vi "osciloscope-4-chan.vi"(0 "COM Port":refnum<visa-resource-name>, 5 "Baud Rate (BPS)":u32=9600, 7 "Sampling Frequency (Hz)":sgl, 9 "Refresh Button":bool, 11 "Stop Button":bool, 12 "Time Domain (Block Size)":u16(knob) scale=4.0..10.0, 13 "Frequency Domain (Block Size)":u16(knob) scale=4.0..10.0, 14 "Decimation Factor":u8=1 min=1 max=100) -> (4 "Time Domain":waveform(dbl)[](graph), 6 "Frequency Domain":cluster{"f0":dbl, "df":dbl, "magnitude":dbl[]}[](graph))   [LabVIEW 2023]
uses:
  <vilib>/Analysis/2dsp.llb/Decimate (single shot, DBL).vi
  <vilib>/Instr/_visa.llb/VISA Configure Serial Port (Instr).vi
  <vilib>/express/express analysis/Spectral/Block/exnSpectralBlock spectral measurements peak poly.vi
  <vilib>/express/express analysis/Spectral/Block/exnSpectralBlock spectral measurements peak WFM.vi
  <vilib>/express/express analysis/Spectral/XNode/ExpressSpectralMeasurementsBlockNode.xnode
  <vilib>/Analysis/NI_AALPro.lvlib
panel:
  out "Frerquency Domain Indicator":u32
  out "Time Domain Indicator":u32
  # "4-CHANNEL OSCILOSCOPE"
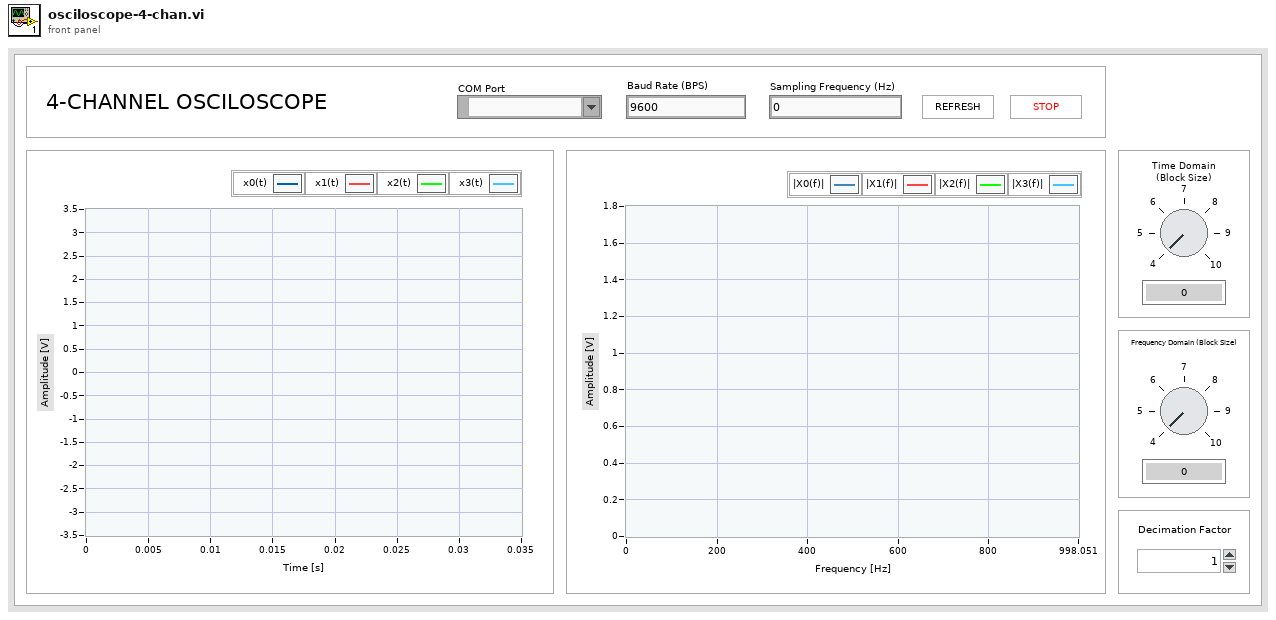
[diagram p1: front panel]
types:
  T1 = cluster{"averaging mode":u16, "weighting mode":u16, "number of averages":u32}
  T2 = cluster{"dB On (F)":bool, "unwrap phase (F)":bool, "convert to degree (F)":bool}
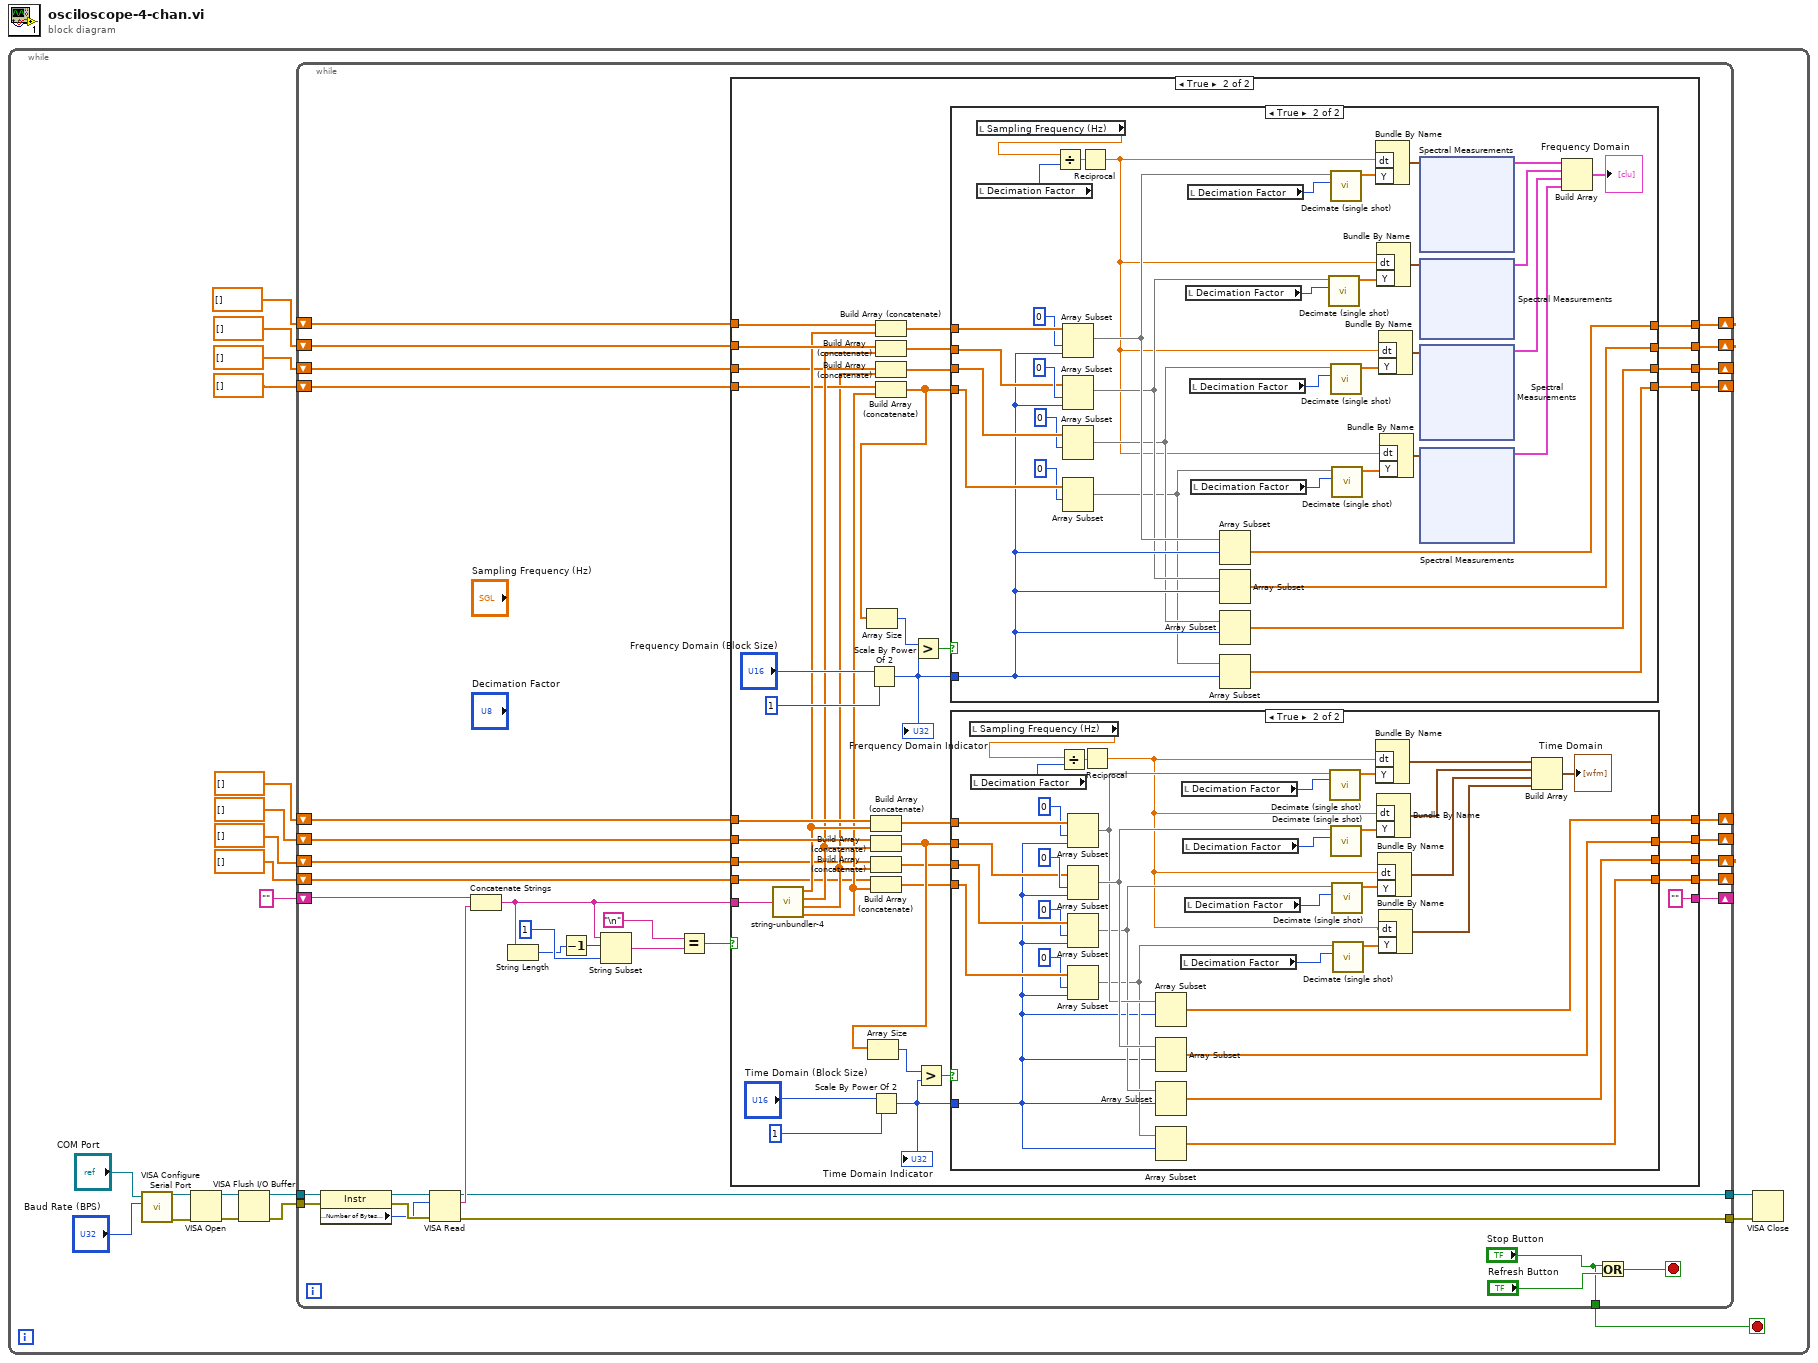
[diagram p0: block diagram]
diagram:
  n1 = while {
    stop <- w9 stop-if-true
    n2 = call-poly "VISA Configure Serial Port"("VISA resource name"="COM Port", "baud rate (9600)"="Baud Rate (BPS)") -> ("VISA resource name out"=w18:refnum<visa-resource-name>, "error out"=w19:errorcluster)  [unwired: 12 in]
    n3 = VISA Open(error in (no error)=w19, VISA resource name=w18) -> (VISA resource name=w17:refnum<visa-resource-name>, error out=w16:errorcluster)  [unwired: 3 in]
    n4 = VISA Flush I/O Buffer(VISA resource name=w17, error in (no error)=w16) -> (VISA resource name out=w20:refnum<visa-resource-name>, error out=w13:errorcluster)  [unwired: 1 in]
    n5 = while {
      tunnel: w20 -> [w56]
      tunnel: w13 -> [w55]
      tunnel: [w36] -> w12
      tunnel: [w37] -> w11
      shift-right: [w49] -> _
      shift-left: "" -> [w50]
      shift-right: [w39] -> _
      shift-left: dbl[] [] -> [w40]
      shift-right: [w38] -> _
      shift-left: dbl[] [] -> [w41]
      shift-right: [w33] -> _
      shift-left: dbl[] [] -> [w35]
      shift-right: [w32] -> _
      shift-left: dbl[] [] -> [w34]
      tunnel: ["Stop Button"] -> w9
      shift-right: [w28] -> _
      shift-left: dbl[] [] -> [w26]
      shift-right: [w27] -> _
      shift-left: dbl[] [] -> [w25]
      shift-right: [w24] -> _
      shift-left: dbl[] [] -> [w22]
      shift-right: [w23] -> _
      shift-left: dbl[] [] -> [w21]
      stop <- w31 stop-if-true
      n6 = property class="Instr"(reference=w56, error in=w55) -> (reference out=w54:refnum<visa-resource-name>, error out=w53:errorcluster, "Serial Settings:Number of Bytes at Serial Port"=w52:u32)
      n7 = VISA Read(VISA resource name=w54, byte count=w52, error in (no error)=w53) -> (VISA resource name out=w37:refnum<visa-resource-name>, read buffer=w51:string, error out=w36:errorcluster)  [unwired: 1 out]
      n8 = Concatenate Strings(w50, w51) -> (w47:string)
      n9 = String Length(string=w47) -> (length=w45:i32)
      n10 = Decrement(x=w45) -> (x-1=w46:i32)
      n11 = String Subset(string=w47, offset (0)=w46, length (rest)=1 ("length (rest)")) -> (substring=w43:string)
      n12 = Equal?(x="\n", y=w43) -> (x = y?=w42:bool)
      n13 = case shown="True" w42 {
        tunnel: w41 -> [w64 w104]
        tunnel: w47 -> [w65 w81]
        tunnel: [w65 ""] -> w49
        tunnel: w40 -> [w63 w102]
        tunnel: [w63 w99] -> w39
        tunnel: [w64 w100] -> w38
        tunnel: w35 -> [w62 w96]
        tunnel: w34 -> [w61 w95]
        tunnel: [w62 w94] -> w33
        tunnel: [w61 w93] -> w32
        tunnel: [w60 w78] -> w28
        tunnel: [w59 w77] -> w27
        tunnel: w26 -> [w60 w76]
        tunnel: w25 -> [w59 w75]
        tunnel: [w58 w72] -> w24
        tunnel: [w57 w71] -> w23
        tunnel: w22 -> [w58 w68]
        tunnel: w21 -> [w57 w67]
        frame False {
        }
        frame True {
          n14 = call "string-unbundler-4.vi"("String"=w81) -> ("Array 1"=w80:dbl[], "Array 2"=w79:dbl[], "Array 3"=w74:dbl[], "Array 4"=w73:dbl[])
          n15 = Scale By Power Of 2(n="Frequency Domain (Block Size)", x=u32 1) -> (x*2^n=w87:u32)
          "Frerquency Domain Indicator" <- w87
          n16 = Build Array (concatenate)(w104, w80) -> (w92:dbl[])
          n17 = Build Array (concatenate)(w102, w79) -> (w98:dbl[])
          n18 = Array Size(array=w98) -> (size(s)=w105:i32)
          n19 = Build Array (concatenate)(w68, w74) -> (w70:dbl[])
          n20 = Build Array (concatenate)(w67, w73) -> (w69:dbl[])
          n21 = Scale By Power Of 2(n="Time Domain (Block Size)", x=u32 1) -> (x*2^n=w84:u32)
          "Time Domain Indicator" <- w84
          n22 = Build Array (concatenate)(w96, w80) -> (w97:dbl[])
          n23 = Build Array (concatenate)(w95, w79) -> (w90:dbl[])
          n24 = Build Array (concatenate)(w76, w74) -> (w82:dbl[])
          n25 = Build Array (concatenate)(w75, w73) -> (w66:dbl[])
          n26 = Array Size(array=w66) -> (size(s)=w89:i32)
          n27 = Greater?(x=w89, y=w87) -> (0:w91:bool)
          n28 = Greater?(x=w105, y=w84) -> (0:w101:bool)
          n29 = case shown="True" w91 {
            tunnel: w97 -> [w109 w147]
            tunnel: w90 -> [w108 w144]
            tunnel: w87 -> [_ w123]
            tunnel: [w109 w143] -> w94
            tunnel: [w108 w142] -> w93
            tunnel: w82 -> [w107 w127]
            tunnel: w66 -> [w106 w125]
            tunnel: [w107 w112] -> w78
            tunnel: [w106 w111] -> w77
            frame False {
            }
            frame True {
              n30 = local read "Sampling Frequency (Hz)"() -> (w132:sgl)
              n31 = local read "Decimation Factor"() -> (w133:u8)
              n32 = Divide(x=w132, y=w133) -> (x/y=w134:sgl)
              n33 = Array Subset(array=w147, index=0, length=w123) -> (w116:dbl[])
              n34 = Array Subset(array=w144, index=0, length=w123) -> (w115:dbl[])
              n35 = Array Subset(array=w127, index=0) -> (w114:dbl[])  [unwired: 1 in]
              n36 = Array Subset(array=w125, index=0) -> (w113:dbl[])  [unwired: 1 in]
              n37 = Reciprocal(x=w134) -> (1/x=w110:sgl)
              n38 = local read "Decimation Factor"() -> (w130:u8)
              n39 = local read "Decimation Factor"() -> (w131:u8)
              n40 = local read "Decimation Factor"() -> (w118:u8)
              n41 = local read "Decimation Factor"() -> (w117:u8)
              n42 = Array Subset(array=w116, index=w123) -> (w143:dbl[])  [unwired: 1 in]
              n43 = Array Subset(array=w115, index=w123) -> (w142:dbl[])  [unwired: 1 in]
              n44 = Array Subset(array=w114, index=w123) -> (w112:dbl[])  [unwired: 1 in]
              n45 = Array Subset(array=w113, index=w123) -> (w111:dbl[])  [unwired: 1 in]
              n46 = call-poly <vilib>:"Decimate (single shot).vi"("decimating factor"=w130, "X"=w115) -> ("Decimated Array"=w136:dbl[])  [unwired: 8 in, 1 out]
              n47 = call-poly <vilib>:"Decimate (single shot).vi"("decimating factor"=w131, "X"=w116) -> ("Decimated Array"=w135:dbl[])  [unwired: 8 in, 1 out]
              n48 = call-poly <vilib>:"Decimate (single shot).vi"("decimating factor"=w118, "X"=w114) -> ("Decimated Array"=w120:dbl[])  [unwired: 8 in, 1 out]
              n49 = call-poly <vilib>:"Decimate (single shot).vi"("decimating factor"=w117, "X"=w113) -> ("Decimated Array"=w119:dbl[])  [unwired: 8 in, 1 out]
              n50 = Bundle By Name("dt"=w110, "Y"=w135) -> (w137:waveform(dbl))  [unwired: 1 in]
              n51 = Bundle By Name("dt"=w110, "Y"=w136) -> (w138:waveform(dbl))  [unwired: 1 in]
              n52 = Bundle By Name("dt"=w110, "Y"=w120) -> (w121:waveform(dbl))  [unwired: 1 in]
              n53 = Bundle By Name("dt"=w110, "Y"=w119) -> (w122:waveform(dbl))  [unwired: 1 in]
              n54 = xnode "Spectral Measurements"("Signals"=w137) -> ("FFT - (Peak)"=w139:cluster{"f0":dbl, "df":dbl, "magnitude":dbl[]})  [unwired: 1 in, 2 out]
              n55 = xnode "Spectral Measurements"("Signals"=w138) -> ("FFT - (Peak)"=w140:cluster{"f0":dbl, "df":dbl, "magnitude":dbl[]})  [unwired: 1 in, 2 out]
              n56 = xnode "Spectral Measurements"("Signals"=w121) -> ("FFT - (Peak)"=w129:cluster{"f0":dbl, "df":dbl, "magnitude":dbl[]})  [unwired: 1 in, 2 out]
              n57 = xnode "Spectral Measurements"("Signals"=w122) -> ("FFT - (Peak)"=w128:cluster{"f0":dbl, "df":dbl, "magnitude":dbl[]})  [unwired: 1 in, 2 out]
              n58 = Build Array(w139, w140, w129, w128) -> (→"Frequency Domain":cluster{"f0":dbl, "df":dbl, "magnitude":dbl[]}[])
            }
          }
          n59 = case shown="True" w101 {
            tunnel: w92 -> [w191 w225]
            tunnel: w98 -> [w190 w223]
            tunnel: w84 -> [_ w195]
            tunnel: [w191 w219] -> w100
            tunnel: [w190 w218] -> w99
            tunnel: [w188 w201] -> w71
            tunnel: [w189 w200] -> w72
            tunnel: w70 -> [w189 w199]
            tunnel: w69 -> [w188 w198]
            frame False {
            }
            frame True {
              n60 = local read "Sampling Frequency (Hz)"() -> (w211:sgl)
              n61 = local read "Decimation Factor"() -> (w212:u8)
              n62 = Divide(x=w211, y=w212) -> (x/y=w210:sgl)
              n63 = Array Subset(array=w225, index=0, length=w195) -> (w215:dbl[])
              n64 = Array Subset(array=w223, index=0, length=w195) -> (w217:dbl[])
              n65 = Array Subset(array=w199, index=0, length=w195) -> (w203:dbl[])
              n66 = Array Subset(array=w198, index=0, length=w195) -> (w202:dbl[])
              n67 = Reciprocal(x=w210) -> (1/x=w192:sgl)
              n68 = Array Subset(array=w215, index=w195) -> (w219:dbl[])  [unwired: 1 in]
              n69 = Array Subset(array=w217, index=w195) -> (w218:dbl[])  [unwired: 1 in]
              n70 = Array Subset(array=w203, index=w195) -> (w200:dbl[])  [unwired: 1 in]
              n71 = Array Subset(array=w202, index=w195) -> (w201:dbl[])  [unwired: 1 in]
              n72 = local read "Decimation Factor"() -> (w193:u8)
              n73 = local read "Decimation Factor"() -> (w209:u8)
              n74 = local read "Decimation Factor"() -> (w208:u8)
              n75 = local read "Decimation Factor"() -> (w194:u8)
              n76 = call-poly <vilib>:"Decimate (single shot).vi"("decimating factor"=w209, "X"=w215) -> ("Decimated Array"=w214:dbl[])  [unwired: 8 in, 1 out]
              n77 = call-poly <vilib>:"Decimate (single shot).vi"("decimating factor"=w208, "X"=w217) -> ("Decimated Array"=w216:dbl[])  [unwired: 8 in, 1 out]
              n78 = call-poly <vilib>:"Decimate (single shot).vi"("decimating factor"=w194, "X"=w203) -> ("Decimated Array"=w206:dbl[])  [unwired: 8 in, 1 out]
              n79 = call-poly <vilib>:"Decimate (single shot).vi"("decimating factor"=w193, "X"=w202) -> ("Decimated Array"=w207:dbl[])  [unwired: 8 in, 1 out]
              n80 = Bundle By Name("dt"=w192, "Y"=w214) -> (w220:waveform(dbl))  [unwired: 1 in]
              n81 = Bundle By Name("dt"=w192, "Y"=w216) -> (w221:waveform(dbl))  [unwired: 1 in]
              n82 = Bundle By Name("dt"=w192, "Y"=w206) -> (w205:waveform(dbl))  [unwired: 1 in]
              n83 = Bundle By Name("dt"=w192, "Y"=w207) -> (w204:waveform(dbl))  [unwired: 1 in]
              n84 = Build Array(w220, w221, w205, w204) -> (→"Time Domain":waveform(dbl)[])
            }
          }
        }
      }
      n85 = Or(x="Stop Button", y="Refresh Button") -> (x .or. y?=w31:bool)
    }
    n86 = VISA Close(VISA resource name=w11, error in (no error)=w12) -> ()  [unwired: 1 out]
  }
